vi "add SR830(SubVI).vi"(6 "字符串":string, 8 "model":string="SR830", 9 "6221":bool) -> (0 "连接的字符串":string, 3 "ok or cancel":bool=TRUE)   [LabVIEW 2019, in "Add Seq.lvlib"]
uses:
  Add Seq.lvlib
  lib/Keithley 622x/Configure/6221 Wave/Typedefs/KE6221 -- Wave Sine Wave Params.ctl
  lib/Keithley 622x/Configure/6221 Wave/Low Level/Typedefs/KE6221 -- Wave Frequency.ctl
  lib/Keithley 622x/Configure/6221 Wave/Low Level/Typedefs/KE6221 -- Wave Amplitude.ctl
  lib/Keithley 622x/Configure/Source/Typedefs/KE622x -- Current Level.ctl
  lib/Keithley 622x/Configure/6221 Wave/Low Level/Typedefs/KE6221 -- Wave Ranging Mode.ctl
  lib/Keithley 622x/Configure/Source/Typedefs/KE622x -- Current Ranges.ctl
  lib/Keithley 622x/Configure/6221 Wave/Low Level/Typedefs/KE6221 -- Wave Playback Mode.ctl
  lib/Keithley 622x/Configure/6221 Wave/Low Level/Typedefs/KE6221 -- Wave Playback Time.ctl
  lib/Keithley 622x/Configure/6221 Wave/Low Level/Typedefs/KE6221 -- Wave Playback Num Cycles.ctl
  lib/Keithley 622x/Configure/6221 Wave/Low Level/Typedefs/KE6221 -- Wave Phase Marker.ctl
  lib/Keithley 622x/Configure/Trigger/Low Level/Typedefs/KE622x -- Trig Link Line.ctl
  SubVI.lvlib
  lib/Keithley 622x/Keithley 622x.lvlib
panel:
  in  "6221(SR830做源可忽略）":T12={"Sine Wave Params In"={"Frequency (Hz)"=1000.0, "Amplitude (A)"=0.001, "Offset (A)"=0.0, "Ranging Mode"=enum."Best", "Fixed Range"=enum."2mA", "Playback Mode"=enum."Time", "Time (s)"=999999.999, "Num Cycles"=1.0, "Phase\nMarker?"=FALSE, "Phase Marker (deg)"=180.0, "Trig Link Line"=enum."1"}, "RMS Amplitude (A)"=0.001, "6221 resource"=""} {"RMS Amplitude (A)" min=2e-12 max=0.105 format="%.3p"; "Sine Wave Params In"."Offset (A)" min=-0.105 max=0.105 format="%.4p"; "Sine Wave Params In"."Num Cycles" min=0.001 max=99999999900.0 format="%.3p"; "Sine Wave Params In"."Time (s)" min=1e-07 max=999999.999 format="%.3p"; "Sine Wave Params In"."Phase Marker (deg)" min=0.0 max=360.0 format="%.3f"; "Sine Wave Params In"."Amplitude (A)" min=2e-12 max=0.105 format="%.3p"; "Sine Wave Params In"."Frequency (Hz)" min=0.001 max=100000.0 format="%.3p"}
  in  "同步 3":bool
  in  "同步 2":bool
  in  "同步":bool
  in  "滤波设置 4":T13={"Time Constant "=8, "Low Pass Filter Slope "=1, "Enable Sync Filter "=TRUE} {"Low Pass Filter Slope" items=["6 dB/oct", "12 dB/oct", "18 db/oct", "24 dB/oct"]; "Time Constant" items=["10 us", "30 us", "100 us", "300 us", "1 ms", "3 ms", "10 ms", "30 ms", "100 ms", "300 ms", "1 s", "3 s", "10 s", "30 s", "100 s", "300 s", "1 ks", "3 ks", "10 ks", "30 ks"]}
  in  "滤波设置 3":T13={"Time Constant "=8, "Low Pass Filter Slope "=1, "Enable Sync Filter "=TRUE} {"Low Pass Filter Slope" items=["6 dB/oct", "12 dB/oct", "18 db/oct", "24 dB/oct"]; "Time Constant" items=["10 us", "30 us", "100 us", "300 us", "1 ms", "3 ms", "10 ms", "30 ms", "100 ms", "300 ms", "1 s", "3 s", "10 s", "30 s", "100 s", "300 s", "1 ks", "3 ks", "10 ks", "30 ks"]}
  in  "滤波设置 2":T13={"Time Constant "=8, "Low Pass Filter Slope "=1, "Enable Sync Filter "=TRUE} {"Low Pass Filter Slope" items=["6 dB/oct", "12 dB/oct", "18 db/oct", "24 dB/oct"]; "Time Constant" items=["10 us", "30 us", "100 us", "300 us", "1 ms", "3 ms", "10 ms", "30 ms", "100 ms", "300 ms", "1 s", "3 s", "10 s", "30 s", "100 s", "300 s", "1 ks", "3 ks", "10 ks", "30 ks"]}
  in  "参考信号 4":T14={"Reference Source"=1, "External Reference Trigger  "=0, "Detection Harmonic Number "=1.0, "Manual Phase (Degree)"=0.0, "Auto Phase "=FALSE, "Sine Output Amplitude (V)"=1.0, "Internal Reference Frequency (Hz)"=13.0} {"External Reference Trigger" items=["Sine Zero Crossing", "TTL Rising Edge", "TTL Falling Edge"]; "Reference Source" items=["External", "Internal"]}
  in  "参考信号 3":T14={"Reference Source"=1, "External Reference Trigger  "=0, "Detection Harmonic Number "=1.0, "Manual Phase (Degree)"=0.0, "Auto Phase "=FALSE, "Sine Output Amplitude (V)"=1.0, "Internal Reference Frequency (Hz)"=13.0} {"External Reference Trigger" items=["Sine Zero Crossing", "TTL Rising Edge", "TTL Falling Edge"]; "Reference Source" items=["External", "Internal"]}
  in  "参考信号 2":T14={"Reference Source"=1, "External Reference Trigger  "=0, "Detection Harmonic Number "=1.0, "Manual Phase (Degree)"=0.0, "Auto Phase "=FALSE, "Sine Output Amplitude (V)"=1.0, "Internal Reference Frequency (Hz)"=13.0} {"External Reference Trigger" items=["Sine Zero Crossing", "TTL Rising Edge", "TTL Falling Edge"]; "Reference Source" items=["External", "Internal"]}
  in  "输入信号 4":T15={"Input Notch Filter "=0, "Input Shield Grounding"=0, "Input Coupling "=0, "Input Connection  "=1} {"Input Connection" items=["Single-Ended Voltage", "Differential Voltage", "1 MOhm Current Gain", "100 MOhm Current Gain"]; "Input Coupling" items=["AC", "DC"]; "Input Shield Grounding" items=["Float", "Ground"]; "Input Notch Filter" items=["None", "Line Notch", "2x Line Notch", "Both Notch Filters"]}
  in  "输入信号 3":T15={"Input Notch Filter "=0, "Input Shield Grounding"=0, "Input Coupling "=0, "Input Connection  "=1} {"Input Connection" items=["Single-Ended Voltage", "Differential Voltage", "1 MOhm Current Gain", "100 MOhm Current Gain"]; "Input Coupling" items=["AC", "DC"]; "Input Shield Grounding" items=["Float", "Ground"]; "Input Notch Filter" items=["None", "Line Notch", "2x Line Notch", "Both Notch Filters"]}
  in  "输入信号 2":T15={"Input Notch Filter "=0, "Input Shield Grounding"=0, "Input Coupling "=0, "Input Connection  "=1} {"Input Connection" items=["Single-Ended Voltage", "Differential Voltage", "1 MOhm Current Gain", "100 MOhm Current Gain"]; "Input Coupling" items=["AC", "DC"]; "Input Shield Grounding" items=["Float", "Ground"]; "Input Notch Filter" items=["None", "Line Notch", "2x Line Notch", "Both Notch Filters"]}
  in  "滤波设置":T13={"Time Constant "=8, "Low Pass Filter Slope "=1, "Enable Sync Filter "=TRUE} {"Low Pass Filter Slope" items=["6 dB/oct", "12 dB/oct", "18 db/oct", "24 dB/oct"]; "Time Constant" items=["10 us", "30 us", "100 us", "300 us", "1 ms", "3 ms", "10 ms", "30 ms", "100 ms", "300 ms", "1 s", "3 s", "10 s", "30 s", "100 s", "300 s", "1 ks", "3 ks", "10 ks", "30 ks"]}
  in  "参考信号":T14={"Reference Source"=1, "External Reference Trigger  "=0, "Detection Harmonic Number "=1.0, "Manual Phase (Degree)"=0.0, "Auto Phase "=FALSE, "Sine Output Amplitude (V)"=1.0, "Internal Reference Frequency (Hz)"=13.0} {"External Reference Trigger" items=["Sine Zero Crossing", "TTL Rising Edge", "TTL Falling Edge"]; "Reference Source" items=["External", "Internal"]}
  in  "输入信号":T15={"Input Notch Filter "=0, "Input Shield Grounding"=0, "Input Coupling "=0, "Input Connection  "=1} {"Input Connection" items=["Single-Ended Voltage", "Differential Voltage", "1 MOhm Current Gain", "100 MOhm Current Gain"]; "Input Coupling" items=["AC", "DC"]; "Input Shield Grounding" items=["Float", "Ground"]; "Input Notch Filter" items=["None", "Line Notch", "2x Line Notch", "Both Notch Filters"]}
  in  "仪器设置":T16={"ID Query"=FALSE, "Reset"=FALSE, "VISA 1"="", "VISA 2"="", "VISA 3"="", "VISA 4"="", "Sensitivity 2"=-1, "Sensitivity 1"=-1, "量程"=enum."量程每次测量会判定", "SR830源配合的阻抗（6221做源可忽略）"=0.0, "SR830 2"=FALSE, "SR830 3"=FALSE, "SR830 4"=FALSE, "Sensitivity 3"=-1, "Sensitivity 4"=-1, "source"=0, "SR830 1"=FALSE} {"source" items=["SR830 1", "SR830 2", "SR830 3", "SR830 4", "6221"]; "Sensitivity 4" items=["Auto Gain"=-1, "2 nV/fA"=0, "5 nV/fA"=1, "10 nV/fA"=2, "20 nV/fA"=3, "50 nV/fA"=4, "100 nV/fA"=5, "200 nV/fA"=6, "500 nV/fA"=7, "1 uV/pA"=8, "2 uV/pA"=9, "5 uV/pA"=10, "10 uV/pA"=11, "20 uV/pA"=12, "50 uV/pA"=13, "100 uV/pA"=14, "200 uV/pA"=15, "500 uV/pA"=16, "1 mV/nA"=17, "2 mV/nA"=18, "5 mV/nA"=19, "10 mV/nA"=20, "20 mV/nA"=21, "50 mV/nA"=22, "100 mV/nA"=23, "200 mV/nA"=24, "500 mV/mA"=25, "1 V/uA"=26]; "Sensitivity 3" items=["Auto Gain"=-1, "2 nV/fA"=0, "5 nV/fA"=1, "10 nV/fA"=2, "20 nV/fA"=3, "50 nV/fA"=4, "100 nV/fA"=5, "200 nV/fA"=6, "500 nV/fA"=7, "1 uV/pA"=8, "2 uV/pA"=9, "5 uV/pA"=10, "10 uV/pA"=11, "20 uV/pA"=12, "50 uV/pA"=13, "100 uV/pA"=14, "200 uV/pA"=15, "500 uV/pA"=16, "1 mV/nA"=17, "2 mV/nA"=18, "5 mV/nA"=19, "10 mV/nA"=20, "20 mV/nA"=21, "50 mV/nA"=22, "100 mV/nA"=23, "200 mV/nA"=24, "500 mV/mA"=25, "1 V/uA"=26]; "Sensitivity 1" items=["Auto Gain"=-1, "2 nV/fA"=0, "5 nV/fA"=1, "10 nV/fA"=2, "20 nV/fA"=3, "50 nV/fA"=4, "100 nV/fA"=5, "200 nV/fA"=6, "500 nV/fA"=7, "1 uV/pA"=8, "2 uV/pA"=9, "5 uV/pA"=10, "10 uV/pA"=11, "20 uV/pA"=12, "50 uV/pA"=13, "100 uV/pA"=14, "200 uV/pA"=15, "500 uV/pA"=16, "1 mV/nA"=17, "2 mV/nA"=18, "5 mV/nA"=19, "10 mV/nA"=20, "20 mV/nA"=21, "50 mV/nA"=22, "100 mV/nA"=23, "200 mV/nA"=24, "500 mV/mA"=25, "1 V/uA"=26]; "Sensitivity 2" items=["Auto Gain"=-1, "2 nV/fA"=0, "5 nV/fA"=1, "10 nV/fA"=2, "20 nV/fA"=3, "50 nV/fA"=4, "100 nV/fA"=5, "200 nV/fA"=6, "500 nV/fA"=7, "1 uV/pA"=8, "2 uV/pA"=9, "5 uV/pA"=10, "10 uV/pA"=11, "20 uV/pA"=12, "50 uV/pA"=13, "100 uV/pA"=14, "200 uV/pA"=15, "500 uV/pA"=16, "1 mV/nA"=17, "2 mV/nA"=18, "5 mV/nA"=19, "10 mV/nA"=20, "20 mV/nA"=21, "50 mV/nA"=22, "100 mV/nA"=23, "200 mV/nA"=24, "500 mV/mA"=25, "1 V/uA"=26]}
  out "错误输出":errorcluster
  in  "load":bool
  in  "cancel":bool
  in  "ok":bool
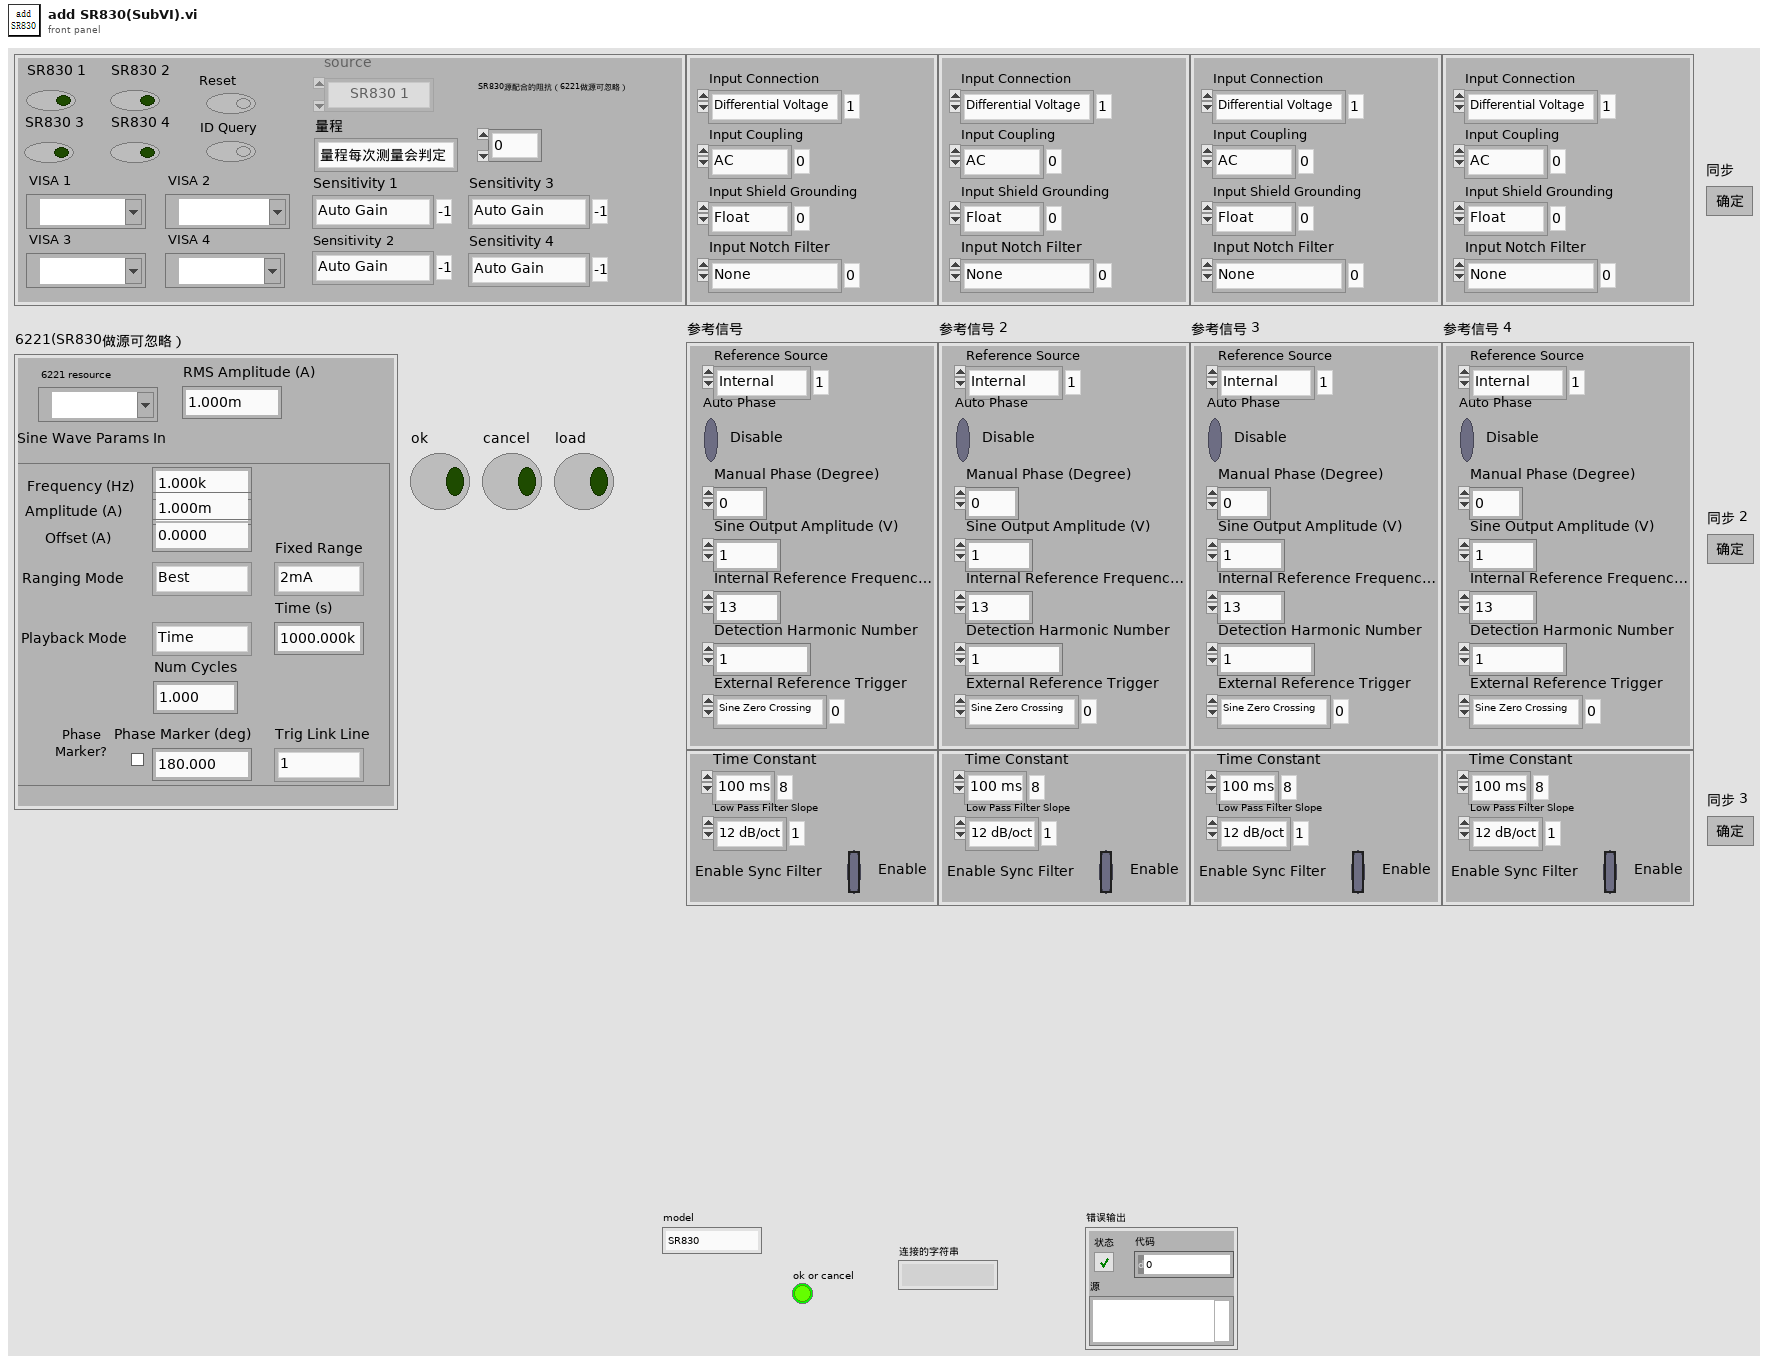
[diagram p1: front panel]
types:
  T1 = typedef "Keithley 622x.lvlib/KE6221 -- Wave Sine Wave Params.ctl" = cluster{"Frequency (Hz)":T2, "Amplitude (A)":T3, "Offset (A)":T4, "Ranging Mode":T5, "Fixed Range":T6, "Playback Mode":T7, "Time (s)":T8, "Num Cycles":T9, "Phase\nMarker?":bool, "Phase Marker (deg)":T10, "Trig Link Line":T11}
  T2 = typedef "Keithley 622x.lvlib/KE6221 -- Wave Frequency.ctl" = dbl
  T3 = typedef "Keithley 622x.lvlib/KE6221 -- Wave Amplitude.ctl" = dbl
  T4 = typedef "Keithley 622x.lvlib/KE622x -- Current Level.ctl" = dbl
  T5 = typedef "Keithley 622x.lvlib/KE6221 -- Wave Ranging Mode.ctl" = enum16{"Best", "Fixed"}
  T6 = typedef "Keithley 622x.lvlib/KE622x -- Current Ranges.ctl" = enum16{"2nA", "20nA", "200nA", "2uA", "20uA", "200uA", "2mA", "20mA", "100mA"}
  T7 = typedef "Keithley 622x.lvlib/KE6221 -- Wave Playback Mode.ctl" = enum16{"Time", "Num Cycles"}
  T8 = typedef "Keithley 622x.lvlib/KE6221 -- Wave Playback Time.ctl" = dbl
  T9 = typedef "Keithley 622x.lvlib/KE6221 -- Wave Playback Num Cycles.ctl" = dbl
  T10 = typedef "Keithley 622x.lvlib/KE6221 -- Wave Phase Marker.ctl" = dbl
  T11 = typedef "Keithley 622x.lvlib/KE622x -- Trig Link Line.ctl" = enum16{"1", "2", "3", "4", "5", "6"}
  T12 = cluster{"Sine Wave Params In":T1, "RMS Amplitude (A)":T3, "6221 resource":refnum<visa-resource-name>}
  T13 = cluster{"Time Constant ":u16, "Low Pass Filter Slope ":u16, "Enable Sync Filter ":bool}
  T14 = cluster{"Reference Source":u16, "External Reference Trigger  ":u16, "Detection Harmonic Number ":dbl, "Manual Phase (Degree)":dbl, "Auto Phase ":bool, "Sine Output Amplitude (V)":dbl, "Internal Reference Frequency (Hz)":dbl}
  T15 = cluster{"Input Notch Filter ":u16, "Input Shield Grounding":u16, "Input Coupling ":u16, "Input Connection  ":u16}
  T16 = cluster{"ID Query":bool, "Reset":bool, "VISA 1":refnum<visa-resource-name>, "VISA 2":refnum<visa-resource-name>, "VISA 3":refnum<visa-resource-name>, "VISA 4":refnum<visa-resource-name>, "Sensitivity 2":i16, "Sensitivity 1":i16, "量程":enum16{"量程每次测量会判定", "量程不变为设定值"}, "SR830源配合的阻抗（6221做源可忽略）":dbl, "SR830 2":bool, "SR830 3":bool, "SR830 4":bool, "Sensitivity 3":i16, "Sensitivity 4":i16, "source":u16, "SR830 1":bool}
  T17 = enum8{"Enabled", "Disabled", "Disabled and Grayed Out"}
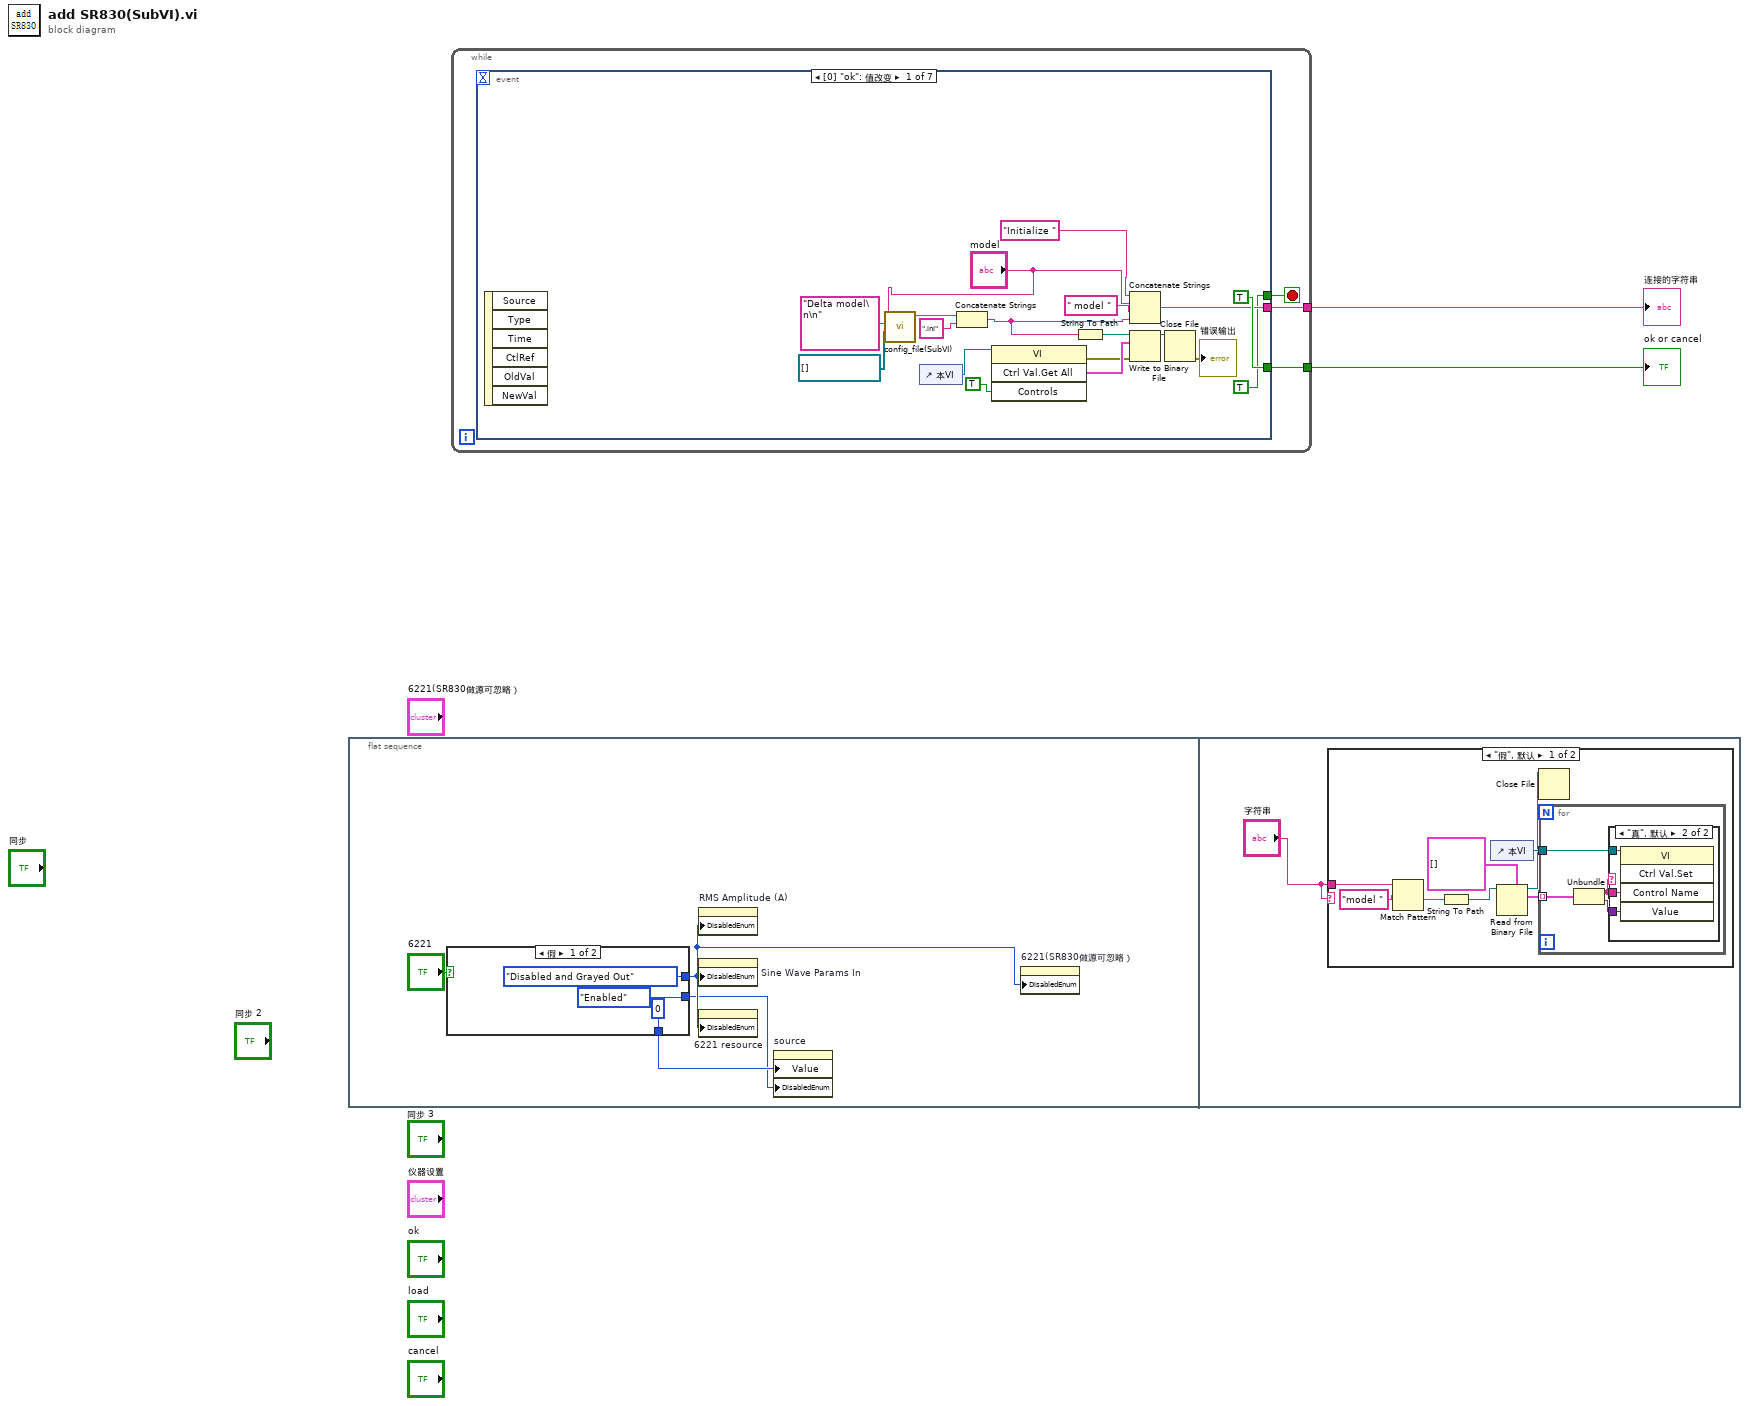
[diagram p0: block diagram]
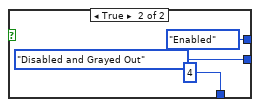
[diagram p2: hidden frame]
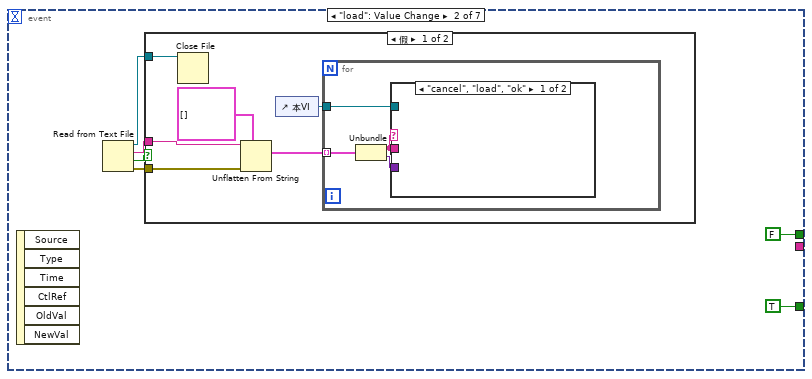
[diagram p5: hidden frame]
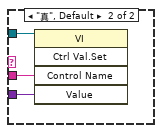
[diagram p6: hidden frame]
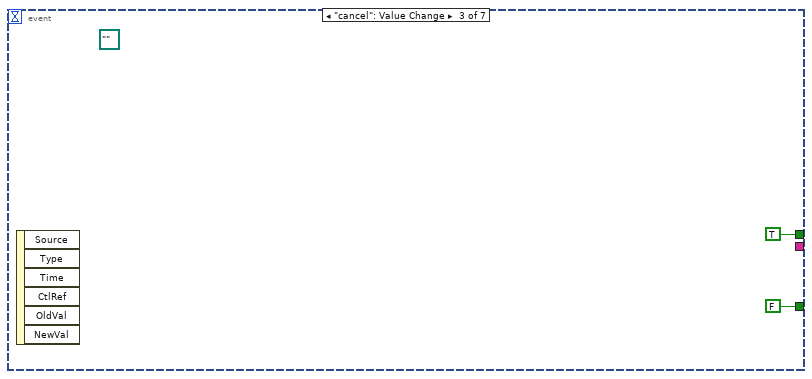
[diagram p8: hidden frame]
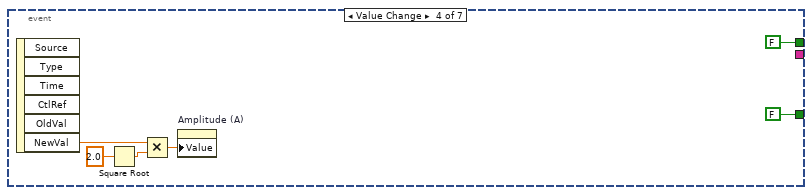
[diagram p9: hidden frame]
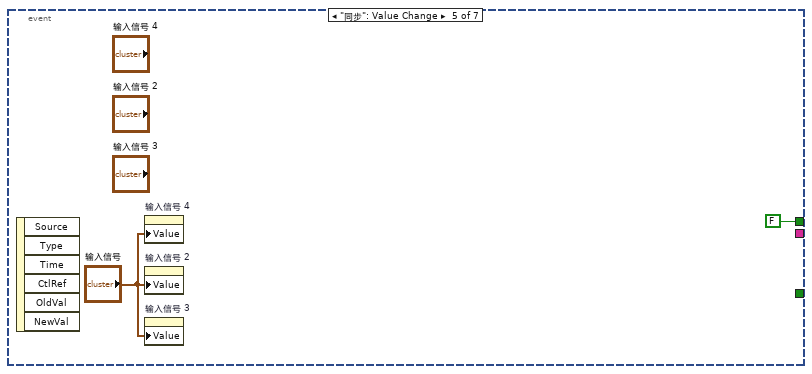
[diagram p10: hidden frame]
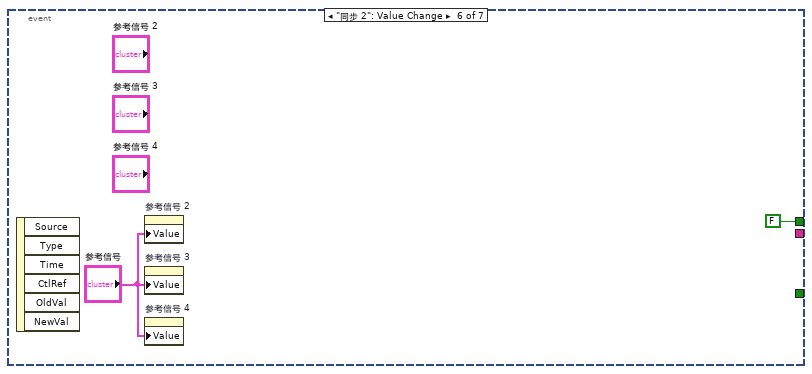
[diagram p11: hidden frame]
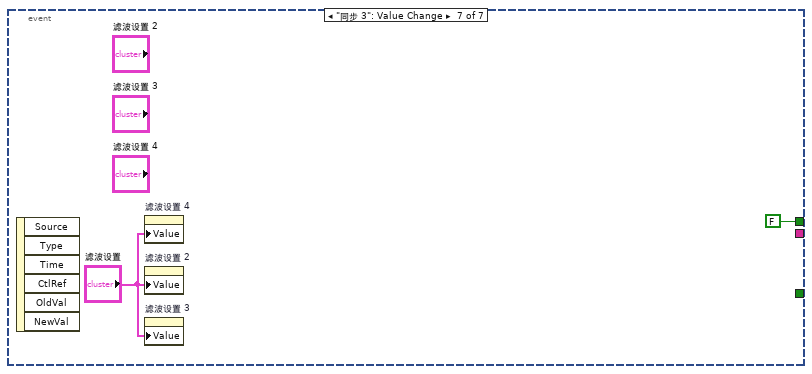
[diagram p12: hidden frame]
diagram:
  n1 = flat-sequence {
    frame #0 {
      n2 = case shown="假" "6221" {
        tunnel: [T17."Disabled and Grayed Out" ("禁用") T17."Enabled" ("禁用")] -> w4
        tunnel: [0 4] -> w5
        tunnel: [T17."Enabled" ("禁用") T17."Disabled and Grayed Out" ("禁用")] -> w3
        frame False {
        }
        frame True {
        }
      }
      n3 = property on="RMS Amplitude (A)" class="DigNum (严格)"("DisabledEnum"=w4) -> ()  [unwired: 2 in, 2 out]
      n4 = property on="Sine Wave Params In" class="Clust (严格)"("DisabledEnum"=w4) -> ()  [unwired: 2 in, 2 out]
      n5 = property on="6221 resource" class="VISAName"("DisabledEnum"=w4) -> ()  [unwired: 2 in, 2 out]
      n6 = property on="source" class="Ring (严格)"("Value"=w5, "DisabledEnum"=w3) -> ()  [unwired: 2 in, 2 out]
      n7 = property on="6221(SR830做源可忽略）" class="Clust (严格)"("DisabledEnum"=w4) -> ()  [unwired: 2 in, 2 out]
    }
    frame #1 {
      n8 = case shown="\"假\", 默认" "字符串" {
        tunnel: "字符串" -> [w21 _]
        frame "假", Default {
          n9 = Match Pattern(string=w21, regular expression="model " ("正则表达式")) -> (after substring=w20:string)  [unwired: 1 in, 3 out]
          n10 = String To Path(string=w20) -> (path=w17:path)
          n11 = control-ref of="本VI"() -> (w18:refnum<vi>)
          n12 = Read from Binary File(5:cluster{"Name":string, "Variant Data":variant}[] [] ("控件值:获取全部"), 11:w17) -> (2:w14:cluster{"Name":string, "Variant Data":variant}[], 3:w16:refnum<file>)  [unwired: 4 in, 2 out]
          n13 = Close File(refnum=w16) -> ()  [unwired: 1 in, 2 out]
          n14 = for {
            tunnel: w14 -> [w25] mode=indexing
            tunnel: w18 -> [w24]
            n15 = Unbundle(w25) -> ("Name"=w22:string, "Variant Data"=w23:variant)
            n16 = case shown="\"真\", 默认" w22 {
              tunnel: w24 -> [_ w28]
              tunnel: w22 -> [_ w27]
              tunnel: w23 -> [_ w26]
              frame "cancel", "load", "ok" {
              }
              frame "真", Default {
                n17 = invoke class="VI" method="Ctrl Val.Set"(reference=w28, "Control Name"=w27, "Value"=w26) -> ()  [unwired: 2 in, 5 out]
              }
            }
          }
        }
        frame "" {
        }
      }
    }
  }
  n18 = while {
    tunnel: [w31] -> w2
    tunnel: [w30] -> w1
    stop <- w29 stop-if-true
    n19 = event shown="[0] \"ok\": 值改变" {
      selector: _ -> [_ _ _ _ _ _ _]
      dyn-events: _ -> [_ _ _ _ _ _ _]
      timeout: _ -> [_ _ _ _ _ _ _]
      tunnel: [TRUE TRUE FALSE FALSE _ _ _] -> w31
      tunnel: [w38 _ _ _ _ _ _] -> w30
      tunnel: [TRUE FALSE TRUE FALSE FALSE FALSE FALSE] -> w29
      event "ok": Value Change {
        n20 = event-data() -> ()  [unwired: 1 in, 6 out]
        n21 = call "config_file(SubVI).vi"("all ref"=refnum<vi>[] [], "文件抬头"="Delta model\n\n", "文件夹名称"="model") -> ("字符串输出"=w44:string)  [unwired: 8 in]
        n22 = control-ref of="本VI"() -> (w47:refnum<vi>)
        n23 = Concatenate Strings(w44, ".ini" ("字符串")) -> (w42:string)
        n24 = invoke class="VI" method="Ctrl Val.Get All"(reference=w47, "Controls"=TRUE ("控件")) -> (error out=w35:errorcluster, "Get All Control Values Variant"=w36:cluster{"Name":string, "Variant Data":variant}[])  [unwired: 2 in, 2 out]
        n25 = String To Path(string=w42) -> (path=w33:path)
        n26 = Concatenate Strings("Initialize " ("字符串"), "model", " model " ("字符串"), w42) -> (w38:string)
        n27 = Write to Binary File(file (use dialog)=w33, data=w36, error in=w35) -> (refnum out=w34:refnum<file>)  [unwired: 3 in, 2 out]
        n28 = Close File(refnum=w34) -> (error out=→"错误输出":errorcluster)  [unwired: 1 in, 1 out]
      }
      event "load": Value Change {
        n29 = event-data() -> ()  [unwired: 1 in, 6 out]
        n30 = Read from Text File() -> (refnum out=w54:refnum<file>, text=w52:string, cancelled=w51:bool, error out=w53:errorcluster)  [unwired: 4 in]
        n31 = case shown="假" w51 {
          tunnel: w54 -> [w61 _]
          tunnel: w53 -> [w59 _]
          tunnel: w52 -> [w58 _]
          frame False {
            n32 = Close File(refnum=w61) -> ()  [unwired: 1 in, 2 out]
            n33 = Unflatten From String(type=cluster{"Name":string, "Variant Data":variant}[] [] ("控件值:获取全部"), binary string=w58, error in (no error)=w59) -> (value=w57:cluster{"Name":string, "Variant Data":variant}[])  [unwired: 2 in, 2 out]
            n34 = control-ref of="本VI"() -> (w56:refnum<vi>)
            n35 = for {
              tunnel: w57 -> [w65] mode=indexing
              tunnel: w56 -> [w64]
              n36 = Unbundle(w65) -> ("Name"=w62:string, "Variant Data"=w63:variant)
              n37 = case shown="\"cancel\", \"load\", \"ok\"" w62 {
                tunnel: w64 -> [_ w68]
                tunnel: w62 -> [_ w67]
                tunnel: w63 -> [_ w66]
                frame "cancel", "load", "ok" {
                }
                frame "真", Default {
                  n38 = invoke class="VI" method="Ctrl Val.Set"(reference=w68, "Control Name"=w67, "Value"=w66) -> ()  [unwired: 2 in, 5 out]
                }
              }
            }
          }
          frame True {
          }
        }
      }
      event "cancel": Value Change {
        (unwired) path "" ("path")
        n39 = event-data() -> ()  [unwired: 1 in, 6 out]
      }
      event Value Change {
        n40 = event-data() -> ("NewVal"=w72:T3)  [unwired: 1 in, 5 out]
        n41 = Square Root(x=2.0) -> (sqrt(x)=w73:dbl)
        n42 = Multiply(x=w72, y=w73) -> (x*y=w71:T3)
        n43 = property on="Amplitude (A)" class="DigNum (严格)"("Value"=w71) -> ()  [unwired: 2 in, 2 out]
      }
      event "同步": Value Change {
        n44 = event-data() -> ()  [unwired: 1 in, 6 out]
        n45 = property on="输入信号 4" class="Clust (严格)"("Value"="输入信号") -> ()  [unwired: 2 in, 2 out]
        n46 = property on="输入信号 2" class="Clust (严格)"("Value"="输入信号") -> ()  [unwired: 2 in, 2 out]
        n47 = property on="输入信号 3" class="Clust (严格)"("Value"="输入信号") -> ()  [unwired: 2 in, 2 out]
      }
      event "同步 2": Value Change {
        n48 = event-data() -> ()  [unwired: 1 in, 6 out]
        n49 = property on="参考信号 2" class="Clust (严格)"("Value"="参考信号") -> ()  [unwired: 2 in, 2 out]
        n50 = property on="参考信号 3" class="Clust (严格)"("Value"="参考信号") -> ()  [unwired: 2 in, 2 out]
        n51 = property on="参考信号 4" class="Clust (严格)"("Value"="参考信号") -> ()  [unwired: 2 in, 2 out]
      }
      event "同步 3": Value Change {
        n52 = event-data() -> ()  [unwired: 1 in, 6 out]
        n53 = property on="滤波设置 4" class="Clust (严格)"("Value"="滤波设置") -> ()  [unwired: 2 in, 2 out]
        n54 = property on="滤波设置 2" class="Clust (严格)"("Value"="滤波设置") -> ()  [unwired: 2 in, 2 out]
        n55 = property on="滤波设置 3" class="Clust (严格)"("Value"="滤波设置") -> ()  [unwired: 2 in, 2 out]
      }
    }
  }
  "ok or cancel" <- w2
  "连接的字符串" <- w1
